vi "Get Task Kind for Preview Channel.vi"(10 "Channel Index":string, 11 "Hardware Configuration in":T1) -> (1 "Task kind":string, 2 "Task name":string)   [LabVIEW 2021, in "Load Frame.lvlib"]
uses:
  Load Frame.lvlib
  Acquisition/Hardware Configuration.ctl
  Acquisition/Channel Settings.ctl
  Acquisition/IO Device.ctl
  Acquisition/Sensor Type.ctl
  Interval Timer/Repeat Interval.ctl
  Interval Timer/Interval Length.ctl
  Interval Timer/Interval Token.ctl
  Acquisition/IO Context.ctl
  Acquisition/IO API.ctl
  Acquisition/Acquisition.lvlib
  Interval Timer/Interval Timer.lvlib
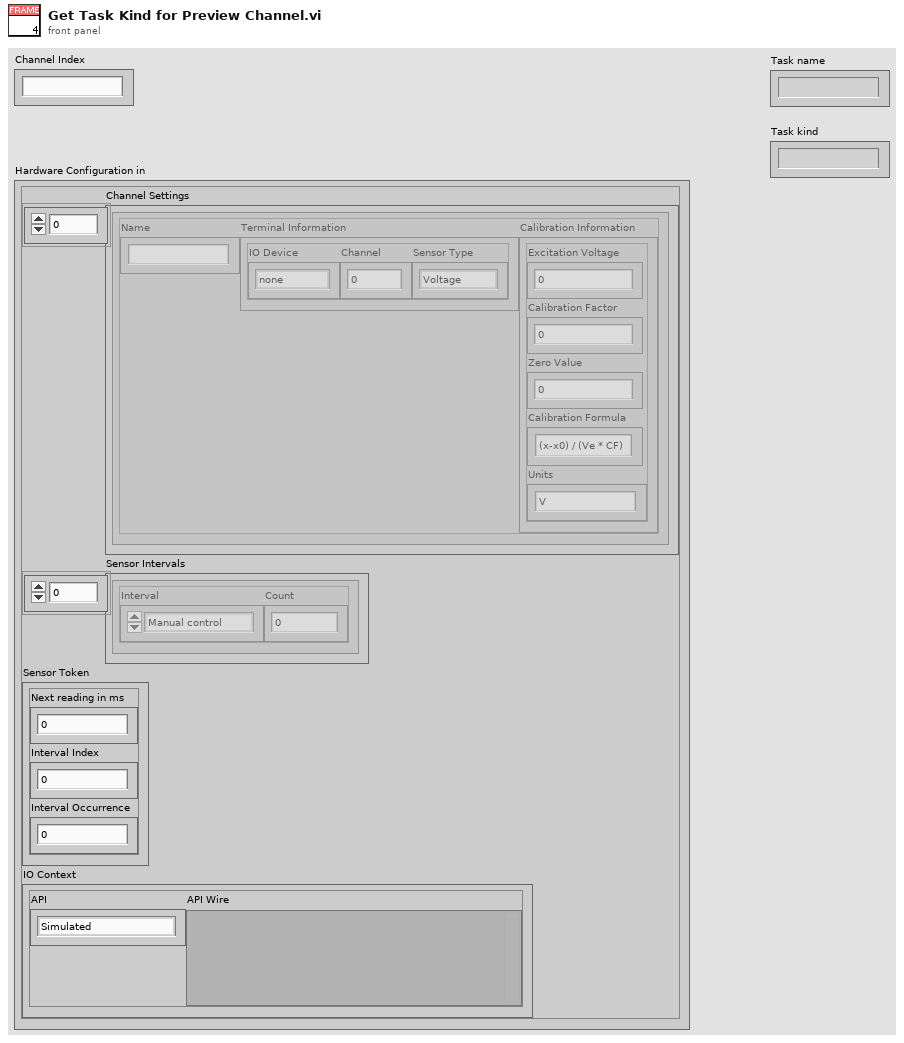
[diagram p1: front panel]
types:
  T1 = typedef "Acquisition.lvlib/Hardware Configuration.ctl" = cluster{"Channel Settings":T2[], "Sensor Intervals":T5[], "Sensor Token":T7, "IO Context":T8}
  T2 = typedef "Acquisition.lvlib/Channel Settings.ctl" = cluster{"Name":string, "Terminal Information":cluster{"IO Device":T3, "Channel":i32, "Sensor Type":T4}, "Calibration Information":cluster{"Excitation Voltage":dbl, "Calibration Factor":dbl, "Zero Value":dbl, "Calibration Formula":string, "Units":string}}
  T3 = typedef "Acquisition.lvlib/IO Device.ctl" = enum16{"none", "9219", "9401"}
  T4 = typedef "Acquisition.lvlib/Sensor Type.ctl" = enum16{"Voltage", "Load", "Pressure", "Encoder"}
  T5 = typedef "Interval Timer.lvlib/Repeat Interval.ctl" = cluster{"Interval":T6, "Count":i32}
  T6 = typedef "Interval Timer.lvlib/Interval Length.ctl" = enum16{"Manual control", "1 second", "10 seconds", "30 seconds", "60 seconds", "600 seconds", "1200 seconds", "3600 seconds"}
  T7 = typedef "Interval Timer.lvlib/Interval Token.ctl" = cluster{"Next reading in ms":u32, "Interval Index":i32, "Interval Occurrence":i32}
  T8 = typedef "Acquisition.lvlib/IO Context.ctl" = cluster{"API":T9, "API Wire":variant}
  T9 = typedef "Acquisition.lvlib/IO API.ctl" = enum16{"Simulated", "DAQmx"}
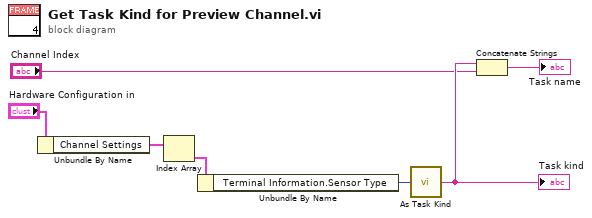
[diagram p0: block diagram]
diagram:
  n1 = Unbundle By Name("Hardware Configuration in") -> ("Channel Settings"=w6:T2[])
  n2 = Index Array(array=w6) -> (element=w5:T2)  [unwired: 1 in]
  n3 = Unbundle By Name(w5) -> ("Terminal Information.Sensor Type"=w4:T4)
  n4 = call "As Task Kind.vi"("Sensor Type"=w4) -> ("DAQmx Task prefix"=w2:string)
  "Task kind" <- w2
  n5 = Concatenate Strings(w2, "Channel Index") -> (→"Task name":string)
